vi "main_impressum.vi"() -> ()   [LabVIEW 2019]
uses:
  <vilib>/Platform/browser.llb/Open URL in Default Browser (string).vi
  <vilib>/Utility/cursorutil.llb/Set Cursor (Icon Pict).vi
panel:
  in  "Stop":bool
  out "String":string
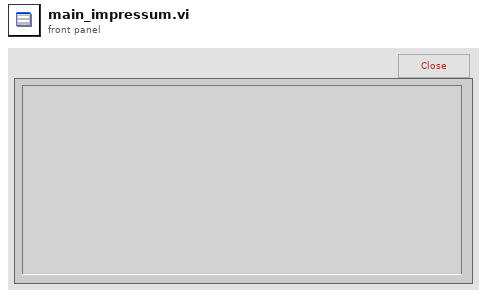
[diagram p1: front panel]
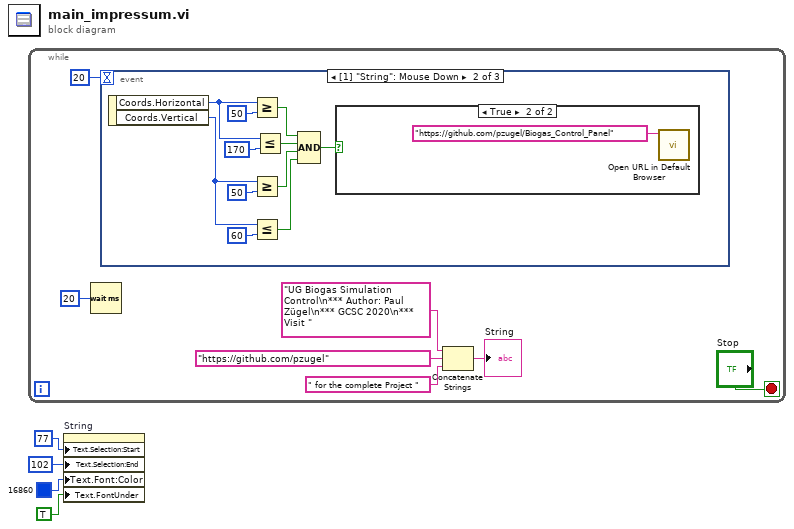
[diagram p0: block diagram]
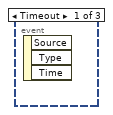
[diagram p2: hidden frame]
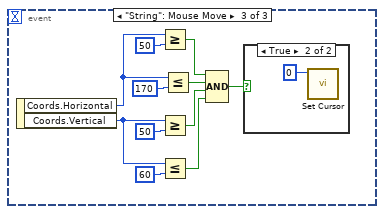
[diagram p4: hidden frame]
diagram:
  n1 = while {
    stop <- "Stop" stop-if-true
    n2 = Wait (ms)(milliseconds to wait=u32 20) -> ()  [unwired: 1 out]
    n3 = event shown="[1] \"String\": Mouse Down" {
      selector: _ -> [_ _ _]
      dyn-events: _ -> [_ _ _]
      timeout: 20 -> [_ _ _]
      event Timeout {
        n4 = event-data() -> ()  [unwired: 1 in, 3 out]
      }
      event "String": Mouse Down {
        n5 = event-data() -> ("Coords.Horizontal"=w19:i32, "Coords.Vertical"=w18:i32)  [unwired: 1 in]
        n6 = Greater Or Equal?(x=w19, y=50 ("x")) -> (x >= y?=w16:bool)
        n7 = Greater Or Equal?(x=w18, y=50 ("x")) -> (x >= y?=w14:bool)
        n8 = Less Or Equal?(x=w18, y=60) -> (x <= y?=w13:bool)
        n9 = Less Or Equal?(x=w19, y=170 ("x")) -> (x <= y?=w15:bool)
        n10 = Compound Arithmetic op=AND(w16, w15, w14, w13) -> (w12:bool)
        n11 = case shown="True" w12 {
          frame False {
          }
          frame True {
            n12 = call-poly <vilib>:"Open URL in Default Browser.vi"("URL"="https://github.com/pzugel/Biogas_Control_Panel") -> ()  [unwired: 5 in, 2 out]
          }
        }
      }
      event "String": Mouse Move {
        n13 = event-data() -> ("Coords.Horizontal"=w25:i32, "Coords.Vertical"=w24:i32)  [unwired: 1 in]
        n14 = Greater Or Equal?(x=w25, y=50 ("x")) -> (x >= y?=w30:bool)
        n15 = Greater Or Equal?(x=w24, y=50 ("x")) -> (x >= y?=w28:bool)
        n16 = Less Or Equal?(x=w24, y=60) -> (x <= y?=w27:bool)
        n17 = Less Or Equal?(x=w25, y=170 ("x")) -> (x <= y?=w29:bool)
        n18 = Compound Arithmetic op=AND(w30, w29, w28, w27) -> (w26:bool)
        n19 = case shown="True" w26 {
          frame False {
          }
          frame True {
            n20 = call-poly <vilib>:"Set Cursor.vi"("icon"=u16 0) -> ()  [unwired: 9 in, 2 out]
          }
        }
      }
    }
    n21 = Concatenate Strings("UG Biogas Simulation Control\n*** Author: Paul Zügel\n*** GCSC 2020\n*** Visit " ("String"), "https://github.com/pzugel" ("URL"), " for the complete Project " ("String")) -> (→"String":string)
  }
  n22 = property on="String" class="Str"("Text.Selection:Start"=u32 77, "Text.Selection:End"=u32 102, "Text.Font:Color"=u32 16860, "Text.FontUnder"=TRUE ("Text.Font:Underline")) -> ()  [unwired: 2 in, 2 out]
